vi "Launcher.vi"() -> ()   [LabVIEW 2020]
panel:
  in  "Refresh":bool
  in  "Run Single Test":bool
  in  "Stop":bool
  in  "Run All Tests":bool
  # "1"
  # "LUnit Test Execution UI"
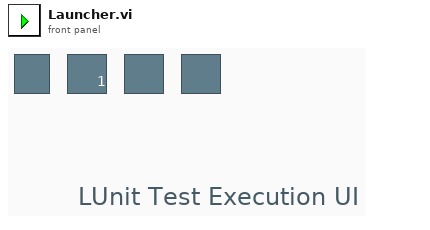
[diagram p1: front panel]
types:
  T1 = enum32{"Invalid", "Standard", "Closed", "Hidden", "Minimized", "Maximized"}
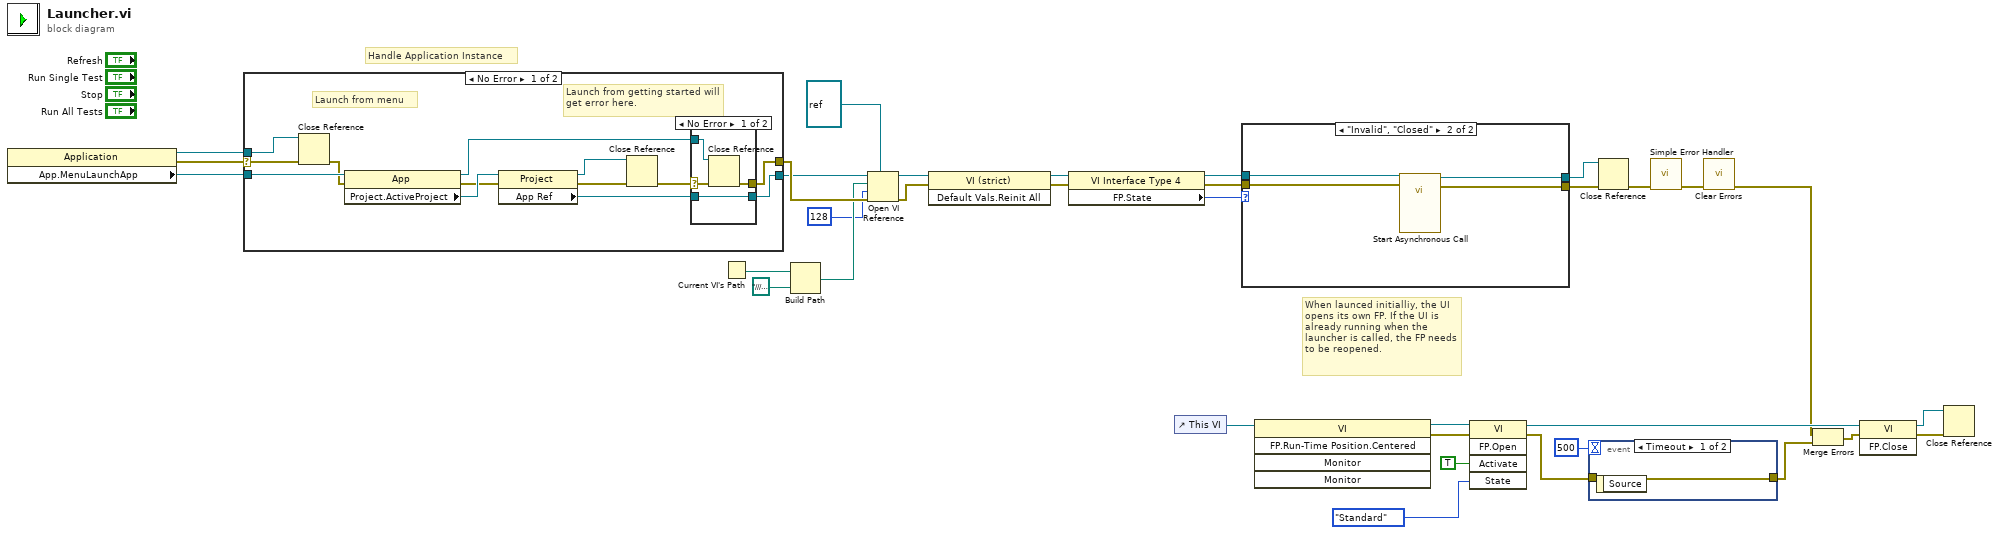
[diagram p0: block diagram]
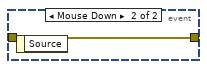
[diagram p2: hidden frame]
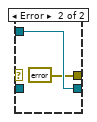
[diagram p3: hidden frame]
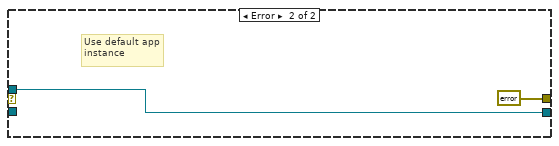
[diagram p4: hidden frame]
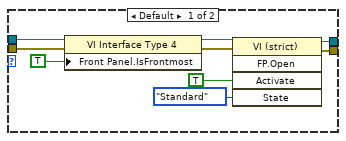
[diagram p5: hidden frame]
diagram:
  # "Handle Application Instance"
  # "When launced initialliy, the UI opens its own FP. If the UI is already running when the launcher is called, the FP needs to be reopened."
  n1 = property class="Application"() -> (reference out=w6:refnum<vi>, error out=w7:errorcluster, "App.MenuLaunchApp"=w8:refnum<vi>)  [unwired: 2 in]
  n2 = case shown="No Error" w7 {
    selector: w7 -> [w46 _]
    tunnel: [w39 w55] -> w12
    tunnel: w8 -> [w44 _]
    tunnel: w6 -> [w47 w55]
    tunnel: [w35 errorcluster {"status"=FALSE, "code"=0, "source"=""} ("error out")] -> w13
    frame No Error {
      # "Launch from getting started will get error here."
      # "Launch from menu"
      n3 = Close Reference(reference=w47, error in (no error)=w46) -> (error out=w43:errorcluster)
      n4 = property class="App"(reference=w44, error in=w43) -> (reference out=w42:refnum<vi>, error out=w40:errorcluster, "Project.ActiveProject"=w45:refnum<vi>)
      n5 = property class="Project"(reference=w45, error in=w40) -> (reference out=w41:refnum<vi>, error out=w37:errorcluster, "App Ref"=w38:refnum<vi>)
      n6 = Close Reference(reference=w41, error in (no error)=w37) -> (error out=w36:errorcluster)
      n7 = case shown="No Error" w36 {
        selector: w36 -> [w50 _]
        tunnel: w42 -> [w51 w53]
        tunnel: [w49 errorcluster {"status"=FALSE, "code"=0, "source"=""} ("error out")] -> w35
        tunnel: [w48 w53] -> w39
        tunnel: w38 -> [w48 _]
        frame No Error {
          n8 = Close Reference(reference=w51, error in (no error)=w50) -> (error out=w49:errorcluster)
        }
        frame Error {
        }
      }
    }
    frame Error {
      # "Use default app instance"
    }
  }
  n9 = Current VI's Path() -> (path=w4:path)
  n10 = Build Path(base path=w4, name or relative path=path "../../../vi.lib/Astemes/LUnit/LUnit User Interface.vi") -> (appended path=w9:path)
  n11 = Open VI Reference(type specifier VI Refnum (for type only)=refnum<vi> refnum, application reference (local)=w12, vi path=w9, options=128, error in (no error)=w13) -> (vi reference=w11:refnum<vi>, error out=w10:errorcluster)  [unwired: 1 in]
  n12 = invoke class="VI (strict)" method="Default Vals.Reinit All"(reference=w11, error in=w10) -> (reference out=w15:refnum<vi>, error out=w14:errorcluster)  [unwired: 1 in, 1 out]
  n13 = property class="VI Interface Type 4"(reference=w15, error in=w14) -> (reference out=w23:refnum<vi>, error out=w22:errorcluster, "FP.State"=w21:T1)
  n14 = control-ref of="This VI"() -> (w34:refnum<vi>)
  n15 = case shown="\"Invalid\", \"Closed\"" w21 {
    tunnel: w23 -> [w62 w68]
    tunnel: w22 -> [w63 w67]
    tunnel: [w57 w66] -> w27
    tunnel: [w56 w65] -> w28
    frame Default {
      n16 = property class="VI Interface Type 4"(reference=w62, error in=w63, "Front Panel.IsFrontmost"=TRUE ("Front Panel Window:Is Frontmost")) -> (reference out=w61:refnum<vi>, error out=w60:errorcluster)
      n17 = invoke class="VI (strict)" method="FP.Open"(reference=w61, error in=w60, "Activate"=TRUE ("Activate?"), "State"=T1."Standard") -> (reference out=w57:refnum<vi>, error out=w56:errorcluster)  [unwired: 1 in, 3 out]
    }
    frame "Invalid", "Closed" {
      n18 = call-by-ref "Start Asynchronous Call"(reference=w68, error in=w67) -> (reference out=w66:refnum<vi>, error out=w65:errorcluster)  [unwired: 12 in]
    }
  }
  n19 = invoke class="VI" method="FP.Run-Time Position.Centered"(reference=w34) -> (reference out=w33:refnum<vi>, error out=w32:errorcluster)  [unwired: 4 in, 3 out]
  n20 = invoke class="VI" method="FP.Open"(reference=w33, error in=w32, "Activate"=TRUE ("Activate?"), "State"=T1."Standard") -> (reference out=w29:refnum<vi>, error out=w18:errorcluster)  [unwired: 1 in, 3 out]
  n21 = event shown="[0] Timeout" {
    selector: _ -> [_ _]
    dyn-events: _ -> [_ _]
    timeout: 500 -> [_ _]
    tunnel: w18 -> [w69 w70]
    tunnel: [w69 w70] -> w16
    event Timeout {
      n22 = event-data() -> ()  [unwired: 1 in, 1 out]
    }
    event Mouse Down {
      n23 = event-data() -> ()  [unwired: 1 in, 1 out]
    }
  }
  n24 = Close Reference(reference=w27, error in (no error)=w28) -> (error out=w25:errorcluster)
  n25 = call <vilib>:"Simple Error Handler.vi"("error in (no error)"=w25) -> ("error out"=w26:errorcluster)  [unwired: 4 in, 4 out]
  n26 = call <vilib>:"Clear Errors.vi"("error in (no error)"=w26) -> ("error out"=w24:errorcluster)  [unwired: 5 in, 1 out]
  n27 = Merge Errors(w24, w16) -> (w17:errorcluster)
  n28 = invoke class="VI" method="FP.Close"(reference=w29, error in=w17) -> (reference out=w19:refnum<vi>, error out=w20:errorcluster)  [unwired: 1 in, 1 out]
  n29 = Close Reference(reference=w19, error in (no error)=w20) -> ()  [unwired: 1 out]
